vi "Clumps to VS Ref Groups.vi"(8 "error in (no error)":errorcluster, 10 "output accesses":T1[](array[typedef]) {"maps"."VS Reference" format="%.0x"}, 11 "input accesses":T6[](array[typedef]) {"Channel Data"."Mapping"."VS Reference" format="%.0x"}) -> (0 "error out":errorcluster, 3 "VS Ref Groups":T9(array[cluster]) {"VS Refs" format="%.0x"})   [LabVIEW 2021]
uses:
  <vilib>/NI VeriStand/Custom Device API/Custom Device Item Ref.ctl
  <vilib>/NI VeriStand/Custom Device API/Custom Device API.lvlib
  <vilib>/NI VeriStand/Custom Device API/Custom Device Channel Type.ctl
  Modbus Master System Explorer.lvlib
  Shared/Controls/Data Model/DataType.ctl
  Shared/Modbus Master Shared.lvlib
  Shared/Controls/Data Model/Mapping.ctl
  Modbus Type.ctl
  Engine/SubVIs/Bulk Data Access.ctl
  Engine/SubVIs/Output Bulk Data Access.ctl
  Shared/Controls/Data Model/Channel.ctl
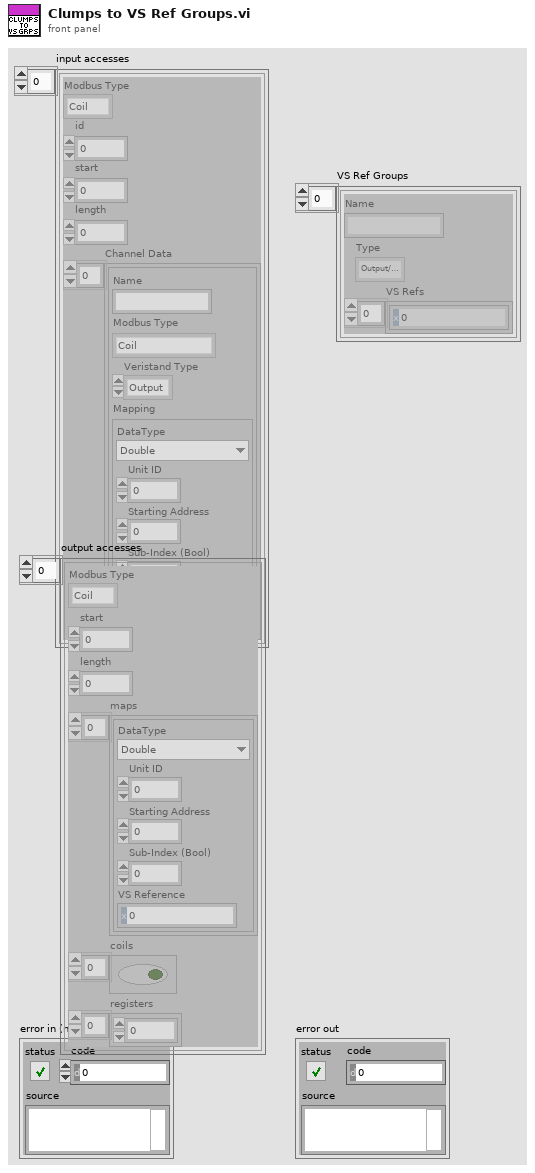
[diagram p1: front panel]
types:
  T1 = typedef "Modbus Master Shared.lvlib/Output Bulk Data Access.ctl" = cluster{"Modbus Type":T2, "start":u16, "length":u16, "maps":T3[], "coils":bool[], "registers":u16[]}
  T2 = typedef "Modbus Master Shared.lvlib/Modbus Type.ctl" = enum16{"Coil", "Discrete Input", "Holding Register", "Input Register"}
  T3 = typedef "Modbus Master Shared.lvlib/Mapping.ctl" = cluster{"DataType":T4, "Unit ID":u8, "Starting Address":u16, "Sub-Index (Bool)":u16, "VS Reference":T5}
  T4 = typedef "Modbus Master Shared.lvlib/DataType.ctl" = enum16{"Double", "Single", "I64", "I32", "I16", "I8", "U64", "U32", "U16", "U8", "Boolean"}
  T5 = typedef "Custom Device API.lvlib/Custom Device Item Ref.ctl" = u64
  T6 = typedef "Modbus Master Shared.lvlib/Bulk Data Access.ctl" = cluster{"Modbus Type":T2, "id":u8, "start":u16, "length":u16, "Channel Data":T7[]}
  T7 = typedef "Modbus Master Shared.lvlib/Channel.ctl" = cluster{"Name":string, "Modbus Type":T2, "Veristand Type":T8, "Mapping":T3}
  T8 = typedef "Custom Device API.lvlib/Custom Device Channel Type.ctl" = enum16{"Input", "Output"}
  T9 = cluster{"Name":string, "Type":enum16{"Output/Write", "Input/Read", "Input/ReadWrite"}, "VS Refs":T5[]}[]
  T10 = cluster{"Name":string, "Type":enum16{"Output/Write", "Input/Read", "Input/ReadWrite"}, "VS Refs":T5[]}
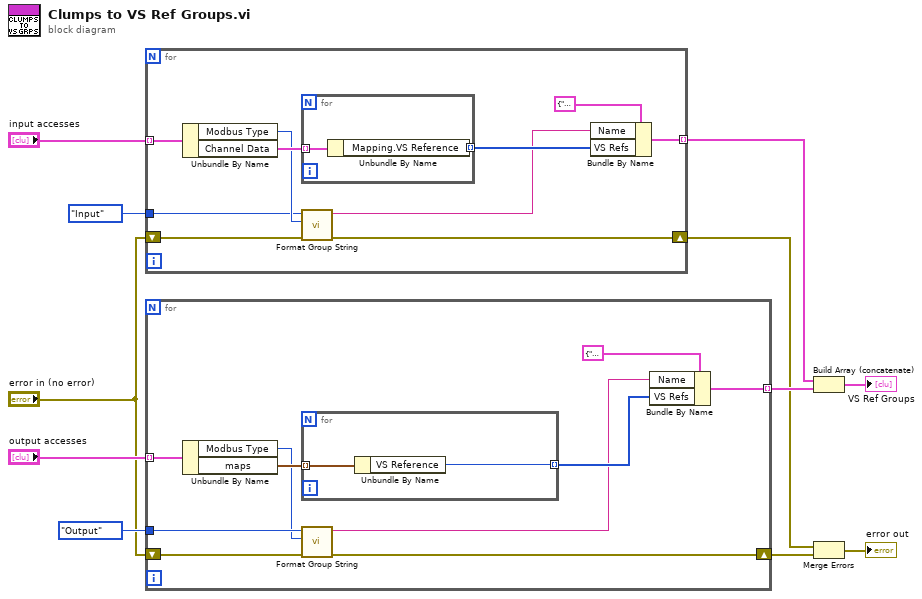
[diagram p0: block diagram]
diagram:
  n1 = for {
    tunnel: "input accesses" -> [w21] mode=indexing
    tunnel: Custom_Device_Channel_Type."Input" ("Veristand Type") -> [w13]
    tunnel: [w17] -> w7 mode=indexing
    shift-right: [w15] -> w3
    shift-left: "error in (no error)" -> [w16]
    n2 = Unbundle By Name(w21) -> ("Modbus Type"=w14:T2, "Channel Data"=w20:T7[])
    n3 = for {
      tunnel: w20 -> [w23] mode=indexing
      tunnel: [w22] -> w18 mode=indexing
      n4 = Unbundle By Name(w23) -> ("Mapping.VS Reference"=w22:T5)
    }
    n5 = call "Format Group String.vi"("error in"=w16, "Modbus Type"=w14, "VS Type"=w13) -> ("error out"=w15:errorcluster, "Group String"=w12:string)  [unwired: 7 in]
    n6 = Bundle By Name(cluster=T10 {"Name"="", "Type"=enum."Input/Read", "VS Refs"=[]} ("Group"), "Name"=w12, "VS Refs"=w18) -> (w17:T10)
  }
  n7 = for {
    tunnel: "output accesses" -> [w33] mode=indexing
    tunnel: Custom_Device_Channel_Type."Output" ("Veristand Type") -> [w28]
    tunnel: [w29] -> w6 mode=indexing
    shift-right: [w24] -> w2
    shift-left: "error in (no error)" -> [w25]
    n8 = Unbundle By Name(w33) -> ("Modbus Type"=w27:T2, "maps"=w32:T3[])
    n9 = for {
      tunnel: w32 -> [w35] mode=indexing
      tunnel: [w34] -> w30 mode=indexing
      n10 = Unbundle By Name(w35) -> ("VS Reference"=w34:T5)
    }
    n11 = call "Format Group String.vi"("error in"=w25, "Modbus Type"=w27, "VS Type"=w28) -> ("error out"=w24:errorcluster, "Group String"=w26:string)  [unwired: 7 in]
    n12 = Bundle By Name(cluster=T10 {"Name"="", "Type"=enum."Output/Write", "VS Refs"=[]} ("Group"), "Name"=w26, "VS Refs"=w30) -> (w29:T10)
  }
  n13 = Build Array (concatenate)(w7, w6) -> (→"VS Ref Groups":T9)
  n14 = Merge Errors(w3, w2) -> (→"error out":errorcluster)
